vi "Get LakeShore 336 Configuration.vi"(8 "error in (no error)":errorcluster, 10 "Config in":T1={"Record Channels"=["A"], "Record raw signal"=FALSE, "Set point"=0.0, "Record heater"=FALSE, "Ramp rate"=0.0, "P"=1.0, "I"=0.0, "D"=60.0, "Control"=enum."Off", "P manual"=0.0, "Output #"=1}, 11 "VISA Resource Name":refnum<visa-resource-name>) -> (0 "error out":errorcluster, 2 "Config out":T1={"Record Channels"=["A"], "Record raw signal"=FALSE, "Set point"=0.0, "Record heater"=FALSE, "Ramp rate"=0.0, "P"=1.0, "I"=0.0, "D"=60.0, "Control"=enum."Off", "P manual"=0.0, "Output #"=0}, 3 "VISA Resource Name Out":refnum<visa-resource-name>)   [LabVIEW 2021]
uses:
  Temperature Controller Driver/T controller configuration.ctl
  Temperature Controller/Controls/Control Mode.ctl
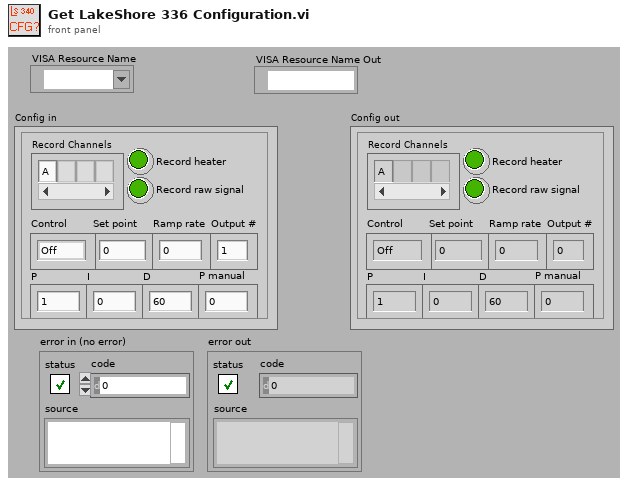
[diagram p1: front panel]
types:
  T1 = typedef "T controller configuration.ctl" = cluster{"Record Channels":string[], "Record raw signal":bool, "Set point":dbl, "Record heater":bool, "Ramp rate":dbl, "P":dbl, "I":dbl, "D":dbl, "Control":T2, "P manual":dbl, "Output #":i32}
  T2 = typedef "Control Mode.ctl" = enum16{"Off", "PID", "Ramp", "Manual", "Table"}
  T3 = typedef "LakeShore340 Mode.ctl" = enum16{"Off", "Closed loop PID", "Zone", "Open loop", "Monitor out", "Warmup supply"}
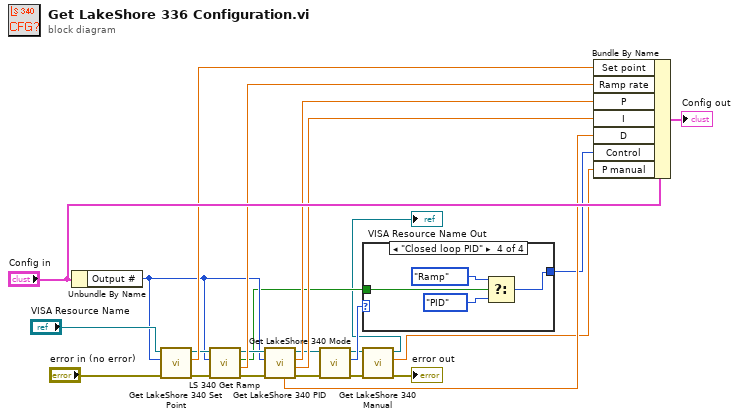
[diagram p0: block diagram]
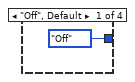
[diagram p2: hidden frame]
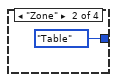
[diagram p3: hidden frame]
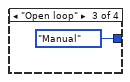
[diagram p4: hidden frame]
diagram:
  n1 = Unbundle By Name("Config in") -> ("Output #"=w14:i32)
  n2 = call "Get LakeShore 340 Set Point.vi"("error in (no error)"="error in (no error)", "Output #"=w14, "VISA Resource Name"="VISA Resource Name") -> ("error out"=w20:errorcluster, "Set point"=w22:dbl, "VISA Resource Name Out"=w21:refnum<visa-resource-name>)  [unwired: 6 in]
  n3 = call "LS 340 Get Ramp.vi"("error in (no error)"=w20, "Output #"=w14, "VISA resource name"=w21) -> ("error out"=w16:errorcluster, "Ramp rate, K/min"=w18:dbl, "Ramp on"=w8:bool, "VISA Resource Name Out"=w15:refnum<visa-resource-name>)  [unwired: 5 in]
  n4 = call "Get LakeShore 340 PID.vi"("error in (no error)"=w16, "Output #"=w14, "VISA Resource Name"=w15) -> ("error out"=w10:errorcluster, "I"=w12:dbl, "P"=w13:dbl, "VISA Resource Name Out"=w6:refnum<visa-resource-name>, "D"=w11:dbl)  [unwired: 4 in]
  n5 = call "Get LakeShore 340 Mode.vi"("error in (no error)"=w10, "VISA Resource Name"=w6) -> ("error out"=w3:errorcluster, "Lake shore mode"=w9:T3, "VISA Resource Name Out"=w5:refnum<visa-resource-name>)  [unwired: 5 in, 2 out]
  n6 = case shown="\"Closed loop PID\"" w9 {
    tunnel: w8 -> [_ _ _ w31]
    tunnel: [Control_Mode."Off" ("Control") Control_Mode."Table" ("Control") Control_Mode."Manual" ("Control") w28] -> w7
    frame "Off", Default {
    }
    frame "Zone" {
    }
    frame "Open loop" {
    }
    frame "Closed loop PID" {
      n7 = Select(t=Control_Mode."Ramp" ("Control"), s=w31, f=Control_Mode."PID" ("Control")) -> (s? t:f=w28:T2)
    }
  }
  n8 = call "Get LakeShore 340 Manual.vi"("error in (no error)"=w3, "VISA Resource Name"=w5) -> ("error out"=→"error out":errorcluster, "Manual otput"=w4:dbl, "VISA Resource Name Out"=→"VISA Resource Name Out":refnum<visa-resource-name>)  [unwired: 7 in]
  n9 = Bundle By Name(cluster="Config in", "Set point"=w22, "Ramp rate"=w18, "P"=w13, "I"=w12, "D"=w11, "Control"=w7, "P manual"=w4) -> (→"Config out":T1)
